vi "ConfigureVelocityController.vi"(0 "axis in":cluster{"keyHandle":u32, "nodeId":u16}={"keyHandle"=0, "nodeId"=1}, 7 "velocity gains":cluster{"p-Gain":u64, "i-Gain":u64}, 11 "error in (no error)":errorcluster) -> (4 "axis out":cluster{"keyHandle":u32, "nodeId":u16}={"keyHandle"=0, "nodeId"=1}, 15 "error out":errorcluster)   [LabVIEW 2017, in "maxonEPOS.lvlib"]
doc: "<B>ConfigureVelocityRegulator</B> writes the velocity regulation gain parameters to the device."
uses:
  Examples/maxonEPOS.lvlib
panel:
  in  "feed forward":T1
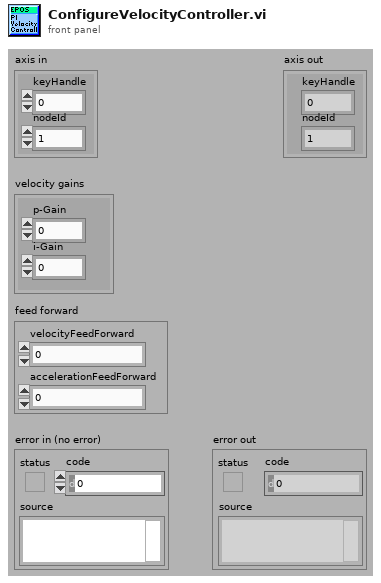
[diagram p1: front panel]
types:
  T1 = cluster{"velocityFeedForward":u64, "accelerationFeedForward":u64}
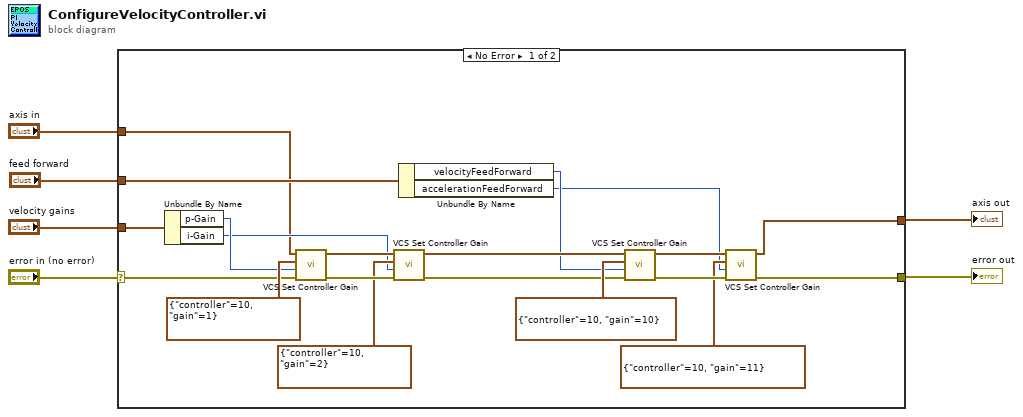
[diagram p0: block diagram]
diagram:
  n1 = case shown="No Error" "error in (no error)" {
    selector: "error in (no error)" -> [w15 w28]
    tunnel: [w16 w28] -> w5
    tunnel: [w8 w27] -> w4
    tunnel: "axis in" -> [w7 w27]
    tunnel: "velocity gains" -> [w14 _]
    tunnel: "feed forward" -> [w11 _]
    frame No Error {
      n2 = Unbundle By Name(w14) -> ("p-Gain"=w13:u64, "i-Gain"=w12:u64)
      n3 = call "VCS Set Controller Gain.vi"("error in (no error)"=w15, "value"=w13, "controller gain"=cluster{"controller":u16, "gain":u16} {"controller"=10, "gain"=1}, "axis in"=w7) -> ("error out"=w26:errorcluster, "axis out"=w23:cluster{"keyHandle":u32, "nodeId":u16})  [unwired: 6 in]
      n4 = call "VCS Set Controller Gain.vi"("error in (no error)"=w26, "value"=w12, "controller gain"=cluster{"controller":u16, "gain":u16} {"controller"=10, "gain"=2}, "axis in"=w23) -> ("error out"=w18:errorcluster, "axis out"=w17:cluster{"keyHandle":u32, "nodeId":u16})  [unwired: 6 in]
      n5 = Unbundle By Name(w11) -> ("velocityFeedForward"=w10:u64, "accelerationFeedForward"=w9:u64)
      n6 = call "VCS Set Controller Gain.vi"("error in (no error)"=w18, "value"=w10, "controller gain"=cluster{"controller":u16, "gain":u16} {"controller"=10, "gain"=10}, "axis in"=w17) -> ("error out"=w25:errorcluster, "axis out"=w24:cluster{"keyHandle":u32, "nodeId":u16})  [unwired: 6 in]
      n7 = call "VCS Set Controller Gain.vi"("error in (no error)"=w25, "value"=w9, "controller gain"=cluster{"controller":u16, "gain":u16} {"controller"=10, "gain"=11}, "axis in"=w24) -> ("error out"=w16:errorcluster, "axis out"=w8:cluster{"keyHandle":u32, "nodeId":u16})  [unwired: 6 in]
    }
    frame Error {
    }
  }
  "error out" <- w5
  "axis out" <- w4
